vi "Connect source-meter(SubIV).vi"(8 "Error In":errorcluster, 11 "Loop data In":T2={"Persistent"={"Last file"=path "", "Last user"="", "Users"=[]}, "Temp handle"={"Connected"=FALSE, "Temp ctrl"={"Gain (P)"=0.0, "Reset (I)"=0.0, "Rate (D)"=0.0, "Stabilization rate"=0.0, "Stabilization delta"=0.0, "Type"=enum."Lake Shore 325", "Custom temp ctrl"={"VISA resource name"=""}, "Lakeshore 325"={"VISA name"="", "Loop"=0, "Heater Range"=1, "Heater Resistance"=0, "Sample sensor"=0, "Fast sensor"=0, "Slow sensor"=0}, "Lakeshore 331"={"VISA name"="", "Loop"=1, "Heater Range"=0, "Sample sensor"=0, "Fast sensor"=0, "Slow sensor"=0}, "Lakeshore 332"={"VISA name"="", "Loop"=1, "Heater Range"=0, "Sample sensor"=0, "Fast sensor"=0, "Slow sensor"=0}, "Lakeshore 335"={"VISA name"="", "Loop"=1, "Sample sensor"=0, "Fast sensor"=0, "Slow sensor"=0, "Heater Range"=0, "Output mode"=enum."Off"}, "Lakeshore 336"={"VISA name"="", "Loop"=1, "Output mode"=enum."Off", "Max current"=1.0, "Heater resistance"=1, "Sample sensor"=1, "Slow sensor"=1, "Fast sensor"=1}}}, "Paths"={"Manual"=path "", "Settings"=path "", "Persistent"=path "", "Work dir."=path ""}, "Settings"={"MFIA"={"Address"="", "Use compensation"=TRUE, "Shut down gracefully"=FALSE}, "Temp ctrl"={"Gain (P)"=0.0, "Reset (I)"=0.0, "Rate (D)"=0.0, "Stabilization rate"=0.0, "Stabilization delta"=0.0, "Type"=enum."Lake Shore 325", "Custom temp ctrl"={"VISA resource name"=""}, "Lakeshore 325"={"VISA name"="", "Loop"=0, "Heater Range"=1, "Heater Resistance"=0, "Sample sensor"=0, "Fast sensor"=0, "Slow sensor"=0}, "Lakeshore 331"={"VISA name"="", "Loop"=1, "Heater Range"=0, "Sample sensor"=0, "Fast sensor"=0, "Slow sensor"=0}, "Lakeshore 332"={"VISA name"="", "Loop"=1, "Heater Range"=0, "Sample sensor"=0, "Fast sensor"=0, "Slow sensor"=0}, "Lakeshore 335"={"VISA name"="", "Loop"=1, "Sample sensor"=0, "Fast sensor"=0, "Slow sensor"=0, "Heater Range"=0, "Output mode"=enum."Off"}, "Lakeshore 336"={"VISA name"="", "Loop"=1, "Output mode"=enum."Off", "Max current"=1.0, "Heater resistance"=1, "Sample sensor"=1, "Slow sensor"=1, "Fast sensor"=1}}, "Source-meter"={"Type"=enum."Custom", "Custom source-meter"={"VISA resource name"=""}, "Keithley 2600"={"VISA name"="", "Ignore ID Query"=FALSE, "SMU"=enum."Channel A"}, "Keithley 2400 Series"={"VISA name"="", "Ignore ID Query"=FALSE}}, "Other"={"Enable OriginLab"=FALSE, "Reader mode"=FALSE, "Auto-save"=FALSE}, "Defaults"={"IV properties"={"T"=0.0, "Vstart"=-0.5, "Vstop"=0.5, "Vpoints"=10.0, "Settling"=0.01, "I limit"=0.1, "Log mapping"=FALSE, "Averaging"=0.0}, "CV properties"={"T"=0.0, "Vstart"=-0.5, "Vstop"=0.5, "Vpoints"=10.0, "Precision"=enum."Normal", "Test signal"=0.01, "Auto I range"=FALSE, "Test frequency"=100000.0, "I range"=-2.0, "V range"=10.0, "Log mapping"=FALSE, "Rel perm"=0.0, "Area"=0.0, "Equivalent circuit model"=0}, "DLTS properties"={"Tstart"=0.0, "Instant start"=FALSE, "Tstop"=0.0, "T rate"=0.0, "Test signal"=0.0, "Test frequency"=0.0, "Bandwidth"=0.0, "Averaging"=0.0, "Vbias"=0.0, "Vpulse"=0.0, "pulse length"=0.0, "Pulse 2"=FALSE, "Vpulse 2"=0.0, "pulse length 2"=0.0, "I range"=-2.0, "V range"=10.0, "Emission rate"=[], "Sampling rate"=0.0, "Acq. delay"=0.0, "Filter order"=0, "Equivalent circuit model"=0}, "LDLTS properties"={"T"=0.0, "Test signal"=0.0, "Test frequency"=0.0, "Bandwidth"=0.0, "Averaging"=0.0, "Vbias"=0.0, "Vpulse"=0.0, "pulse length"=0.0, "Pulse 2"=FALSE, "Vpulse 2"=0.0, "pulse length 2"=0.0, "I range"=-2.0, "V range"=10.0, "Sampling rate"=0.0, "Acq. delay"=0.0, "Sampling time"=0.0, "Filter order"=0, "Equivalent circuit model"=0}}}, "Software version"=0.0, "MFIA handle"={"ziHandle"={"handleValid"=FALSE, "Conn"=0, "Path Prefix"="", "Handle"=0, "Connected"=FALSE, "Clockbase(s)"=0.0}, "Selected device"="", "ziModHandle"={"handleValid"=FALSE, "Conn"=0, "ModHandle"=0, "moduleID"="", "Path Prefix"=""}}, "Source-meter handle"={"Connected"=FALSE, "Source-meter"={"Type"=enum."Keithley 2600", "Custom source-meter"={"VISA resource name"=""}, "Keithley 2600"={"VISA name"="", "Ignore ID Query"=FALSE, "SMU"=enum."Channel A"}, "Keithley 2400 Series"={"VISA name"="", "Ignore ID Query"=FALSE}}}} {"MFIA handle"."ziModHandle"."ModHandle" format="0x%08x"; "MFIA handle"."ziModHandle"."Conn" format="0x%08x"; "MFIA handle"."ziHandle"."Handle" format="0x%08x"; "MFIA handle"."ziHandle"."Conn" format="0x%08x"; "Settings"."Defaults"."LDLTS properties"."Equivalent circuit model" items=["Rp || Cp", "Rs + Cs", "Rs + Ls", "G B", "D Cs", "Q Cs", "D Ls", "Q Ls", "Rp || Lp", "D Cp"]; "Settings"."Defaults"."LDLTS properties"."Filter order" min=0 max=8 step=1; "Settings"."Defaults"."LDLTS properties"."Sampling rate" items=["13k"=13392.857422, "27k"=26785.714844, "54k"=53571.429687, "107k"=107142.859375]; "Settings"."Defaults"."LDLTS properties"."V range" items=["10mV"=0.01, "100mV"=0.1, "1V"=1.0, "10V"=10.0]; "Settings"."Defaults"."LDLTS properties"."I range" items=["100nA"=-7.0, "1µA"=-6.0, "10µA"=-5.0, "100µA"=-4.0, "1mA"=-3.0, "10mA"=-2.0]; "Settings"."Defaults"."DLTS properties"."Equivalent circuit model" items=["Rp || Cp", "Rs + Cs", "Rs + Ls", "G B", "D Cs", "Q Cs", "D Ls", "Q Ls", "Rp || Lp", "D Cp"]; "Settings"."Defaults"."DLTS properties"."Filter order" min=0 max=8 step=1; "Settings"."Defaults"."DLTS properties"."Sampling rate" items=["13k"=13392.857422, "27k"=26785.714844, "54k"=53571.429687, "107k"=107142.859375]; "Settings"."Defaults"."DLTS properties"."V range" items=["10mV"=0.01, "100mV"=0.1, "1V"=1.0, "10V"=10.0]; "Settings"."Defaults"."DLTS properties"."I range" items=["10mV"=0.01, "100mV"=0.1, "1V"=1.0, "10V"=10.0]; "Settings"."Defaults"."CV properties"."Equivalent circuit model" items=["Rp || Cp", "Rs + Cs", "Rs + Ls", "G B", "D Cs", "Q Cs", "D Ls", "Q Ls", "Rp || Lp", "D Cp"]; "Settings"."Defaults"."CV properties"."V range" items=["10mV"=0.01, "100mV"=0.1, "1V"=1.0, "10V"=10.0]; "Settings"."Defaults"."CV properties"."I range" items=["100nA"=-7.0, "1µA"=-6.0, "10µA"=-5.0, "100µA"=-4.0, "1mA"=-3.0, "10mA"=-2.0]; "Settings"."Defaults"."IV properties"."Settling" min=0.0 max=65535.0; "Settings"."Temp ctrl"."Lakeshore 336"."Fast sensor" items=["Sensor A", "Sensor B", "Sensor C", "Sensor D"]; "Settings"."Temp ctrl"."Lakeshore 336"."Slow sensor" items=["Sensor A", "Sensor B", "Sensor C", "Sensor D"]; "Settings"."Temp ctrl"."Lakeshore 336"."Sample sensor" items=["Sensor A", "Sensor B", "Sensor C", "Sensor D"]; "Settings"."Temp ctrl"."Lakeshore 336"."Heater resistance" items=["25 Ohm"=1, "50 Ohm"=2]; "Settings"."Temp ctrl"."Lakeshore 336"."Max current" items=["0.707 A"=0.0, "1 A"=1.0, "1.414 A"=1.414, "2 A"=2.0]; "Settings"."Temp ctrl"."Lakeshore 336"."Loop" items=["Output 1"=1, "Output 2"=2, "Output 3"=3, "Output 4"=4]; "Settings"."Temp ctrl"."Lakeshore 335"."Heater Range" items=["Off", "Low (On)", "Medium", "High"]; "Settings"."Temp ctrl"."Lakeshore 335"."Slow sensor" items=["A", "B"]; "Settings"."Temp ctrl"."Lakeshore 335"."Fast sensor" items=["A", "B"]; "Settings"."Temp ctrl"."Lakeshore 335"."Sample sensor" items=["A", "B"]; "Settings"."Temp ctrl"."Lakeshore 335"."Loop" items=["Loop 1"=1, "Loop 2"=2]; "Settings"."Temp ctrl"."Lakeshore 332"."Slow sensor" items=["A", "B"]; "Settings"."Temp ctrl"."Lakeshore 332"."Fast sensor" items=["A", "B"]; "Settings"."Temp ctrl"."Lakeshore 332"."Sample sensor" items=["A", "B"]; "Settings"."Temp ctrl"."Lakeshore 332"."Heater Range" items=["Off", "Low (0.5W)", "Med (5W)", "High (50W)"]; "Settings"."Temp ctrl"."Lakeshore 332"."Loop" items=["Loop 1", "Loop 2"]; "Settings"."Temp ctrl"."Lakeshore 331"."Slow sensor" items=["A", "B"]; "Settings"."Temp ctrl"."Lakeshore 331"."Fast sensor" items=["A", "B"]; "Settings"."Temp ctrl"."Lakeshore 331"."Sample sensor" items=["A", "B"]; "Settings"."Temp ctrl"."Lakeshore 331"."Heater Range" items=["Off", "Low (0.5W)", "Med (5W)", "High (50W)"]; "Settings"."Temp ctrl"."Lakeshore 331"."Loop" items=["Loop 1", "Loop 2"]; "Settings"."Temp ctrl"."Lakeshore 325"."Slow sensor" items=["A", "B"]; "Settings"."Temp ctrl"."Lakeshore 325"."Fast sensor" items=["A", "B"]; "Settings"."Temp ctrl"."Lakeshore 325"."Sample sensor" items=["A", "B"]; "Settings"."Temp ctrl"."Lakeshore 325"."Heater Resistance" items=["25 Ohm"=1, "50 Ohm"=2]; "Settings"."Temp ctrl"."Lakeshore 325"."Heater Range" items=["Off", "Low (loop 1) or On (loop 2)", "High (loop 1)"]; "Settings"."Temp ctrl"."Lakeshore 325"."Loop" items=["Loop 1"=1, "Loop 2"=2]; "Temp handle"."Temp ctrl"."Lakeshore 336"."Fast sensor" items=["Sensor A", "Sensor B", "Sensor C", "Sensor D"]; "Temp handle"."Temp ctrl"."Lakeshore 336"."Slow sensor" items=["Sensor A", "Sensor B", "Sensor C", "Sensor D"]; "Temp handle"."Temp ctrl"."Lakeshore 336"."Sample sensor" items=["Sensor A", "Sensor B", "Sensor C", "Sensor D"]; "Temp handle"."Temp ctrl"."Lakeshore 336"."Heater resistance" items=["25 Ohm"=1, "50 Ohm"=2]; "Temp handle"."Temp ctrl"."Lakeshore 336"."Max current" items=["0.707 A"=0.0, "1 A"=1.0, "1.414 A"=1.414, "2 A"=2.0]; "Temp handle"."Temp ctrl"."Lakeshore 336"."Loop" items=["Output 1"=1, "Output 2"=2, "Output 3"=3, "Output 4"=4]; "Temp handle"."Temp ctrl"."Lakeshore 335"."Heater Range" items=["Off", "Low (On)", "Medium", "High"]; "Temp handle"."Temp ctrl"."Lakeshore 335"."Slow sensor" items=["A", "B"]; "Temp handle"."Temp ctrl"."Lakeshore 335"."Fast sensor" items=["A", "B"]; "Temp handle"."Temp ctrl"."Lakeshore 335"."Sample sensor" items=["A", "B"]; "Temp handle"."Temp ctrl"."Lakeshore 335"."Loop" items=["Loop 1"=1, "Loop 2"=2]; "Temp handle"."Temp ctrl"."Lakeshore 332"."Slow sensor" items=["A", "B"]; "Temp handle"."Temp ctrl"."Lakeshore 332"."Fast sensor" items=["A", "B"]; "Temp handle"."Temp ctrl"."Lakeshore 332"."Sample sensor" items=["A", "B"]; "Temp handle"."Temp ctrl"."Lakeshore 332"."Heater Range" items=["Off", "Low (0.5W)", "Med (5W)", "High (50W)"]; "Temp handle"."Temp ctrl"."Lakeshore 332"."Loop" items=["Loop 1", "Loop 2"]; "Temp handle"."Temp ctrl"."Lakeshore 331"."Slow sensor" items=["A", "B"]; "Temp handle"."Temp ctrl"."Lakeshore 331"."Fast sensor" items=["A", "B"]; "Temp handle"."Temp ctrl"."Lakeshore 331"."Sample sensor" items=["A", "B"]; "Temp handle"."Temp ctrl"."Lakeshore 331"."Heater Range" items=["Off", "Low (0.5W)", "Med (5W)", "High (50W)"]; "Temp handle"."Temp ctrl"."Lakeshore 331"."Loop" items=["Loop 1", "Loop 2"]; "Temp handle"."Temp ctrl"."Lakeshore 325"."Slow sensor" items=["A", "B"]; "Temp handle"."Temp ctrl"."Lakeshore 325"."Fast sensor" items=["A", "B"]; "Temp handle"."Temp ctrl"."Lakeshore 325"."Sample sensor" items=["A", "B"]; "Temp handle"."Temp ctrl"."Lakeshore 325"."Heater Resistance" items=["25 Ohm"=1, "50 Ohm"=2]; "Temp handle"."Temp ctrl"."Lakeshore 325"."Heater Range" items=["Off", "Low (loop 1) or On (loop 2)", "High (loop 1)"]; "Temp handle"."Temp ctrl"."Lakeshore 325"."Loop" items=["Loop 1"=1, "Loop 2"=2]}) -> (0 "Error Out":errorcluster, 2 "Result":T1(ring), 3 "Loop data Out":T2={"Persistent"={"Last file"=path "", "Last user"="", "Users"=[]}, "Temp handle"={"Connected"=FALSE, "Temp ctrl"={"Gain (P)"=0.0, "Reset (I)"=0.0, "Rate (D)"=0.0, "Stabilization rate"=0.0, "Stabilization delta"=0.0, "Type"=enum."Lake Shore 325", "Custom temp ctrl"={"VISA resource name"=""}, "Lakeshore 325"={"VISA name"="", "Loop"=0, "Heater Range"=1, "Heater Resistance"=0, "Sample sensor"=0, "Fast sensor"=0, "Slow sensor"=0}, "Lakeshore 331"={"VISA name"="", "Loop"=1, "Heater Range"=0, "Sample sensor"=0, "Fast sensor"=0, "Slow sensor"=0}, "Lakeshore 332"={"VISA name"="", "Loop"=1, "Heater Range"=0, "Sample sensor"=0, "Fast sensor"=0, "Slow sensor"=0}, "Lakeshore 335"={"VISA name"="", "Loop"=1, "Sample sensor"=0, "Fast sensor"=0, "Slow sensor"=0, "Heater Range"=0, "Output mode"=enum."Off"}, "Lakeshore 336"={"VISA name"="", "Loop"=1, "Output mode"=enum."Off", "Max current"=1.0, "Heater resistance"=1, "Sample sensor"=1, "Slow sensor"=1, "Fast sensor"=1}}}, "Paths"={"Manual"=path "", "Settings"=path "", "Persistent"=path "", "Work dir."=path ""}, "Settings"={"MFIA"={"Address"="", "Use compensation"=TRUE, "Shut down gracefully"=FALSE}, "Temp ctrl"={"Gain (P)"=0.0, "Reset (I)"=0.0, "Rate (D)"=0.0, "Stabilization rate"=0.0, "Stabilization delta"=0.0, "Type"=enum."Lake Shore 325", "Custom temp ctrl"={"VISA resource name"=""}, "Lakeshore 325"={"VISA name"="", "Loop"=0, "Heater Range"=1, "Heater Resistance"=0, "Sample sensor"=0, "Fast sensor"=0, "Slow sensor"=0}, "Lakeshore 331"={"VISA name"="", "Loop"=1, "Heater Range"=0, "Sample sensor"=0, "Fast sensor"=0, "Slow sensor"=0}, "Lakeshore 332"={"VISA name"="", "Loop"=1, "Heater Range"=0, "Sample sensor"=0, "Fast sensor"=0, "Slow sensor"=0}, "Lakeshore 335"={"VISA name"="", "Loop"=1, "Sample sensor"=0, "Fast sensor"=0, "Slow sensor"=0, "Heater Range"=0, "Output mode"=enum."Off"}, "Lakeshore 336"={"VISA name"="", "Loop"=1, "Output mode"=enum."Off", "Max current"=1.0, "Heater resistance"=1, "Sample sensor"=1, "Slow sensor"=1, "Fast sensor"=1}}, "Source-meter"={"Type"=enum."Custom", "Custom source-meter"={"VISA resource name"=""}, "Keithley 2600"={"VISA name"="", "Ignore ID Query"=FALSE, "SMU"=enum."Channel A"}, "Keithley 2400 Series"={"VISA name"="", "Ignore ID Query"=FALSE}}, "Other"={"Enable OriginLab"=FALSE, "Reader mode"=FALSE, "Auto-save"=FALSE}, "Defaults"={"IV properties"={"T"=0.0, "Vstart"=-0.5, "Vstop"=0.5, "Vpoints"=10.0, "Settling"=0.01, "I limit"=0.1, "Log mapping"=FALSE, "Averaging"=0.0}, "CV properties"={"T"=0.0, "Vstart"=-0.5, "Vstop"=0.5, "Vpoints"=10.0, "Precision"=enum."Normal", "Test signal"=0.01, "Auto I range"=FALSE, "Test frequency"=100000.0, "I range"=-2.0, "V range"=10.0, "Log mapping"=FALSE, "Rel perm"=0.0, "Area"=0.0, "Equivalent circuit model"=0}, "DLTS properties"={"Tstart"=0.0, "Instant start"=FALSE, "Tstop"=0.0, "T rate"=0.0, "Test signal"=0.0, "Test frequency"=0.0, "Bandwidth"=0.0, "Averaging"=0.0, "Vbias"=0.0, "Vpulse"=0.0, "pulse length"=0.0, "Pulse 2"=FALSE, "Vpulse 2"=0.0, "pulse length 2"=0.0, "I range"=-2.0, "V range"=10.0, "Emission rate"=[], "Sampling rate"=0.0, "Acq. delay"=0.0, "Filter order"=0, "Equivalent circuit model"=0}, "LDLTS properties"={"T"=0.0, "Test signal"=0.0, "Test frequency"=0.0, "Bandwidth"=0.0, "Averaging"=0.0, "Vbias"=0.0, "Vpulse"=0.0, "pulse length"=0.0, "Pulse 2"=FALSE, "Vpulse 2"=0.0, "pulse length 2"=0.0, "I range"=-2.0, "V range"=10.0, "Sampling rate"=0.0, "Acq. delay"=0.0, "Sampling time"=0.0, "Filter order"=0, "Equivalent circuit model"=0}}}, "Software version"=0.0, "MFIA handle"={"ziHandle"={"handleValid"=FALSE, "Conn"=0, "Path Prefix"="", "Handle"=0, "Connected"=FALSE, "Clockbase(s)"=0.0}, "Selected device"="", "ziModHandle"={"handleValid"=FALSE, "Conn"=0, "ModHandle"=0, "moduleID"="", "Path Prefix"=""}}, "Source-meter handle"={"Connected"=FALSE, "Source-meter"={"Type"=enum."Keithley 2600", "Custom source-meter"={"VISA resource name"=""}, "Keithley 2600"={"VISA name"="", "Ignore ID Query"=FALSE, "SMU"=enum."Channel A"}, "Keithley 2400 Series"={"VISA name"="", "Ignore ID Query"=FALSE}}}} {"MFIA handle"."ziModHandle"."ModHandle" format="0x%08x"; "MFIA handle"."ziModHandle"."Conn" format="0x%08x"; "MFIA handle"."ziHandle"."Handle" format="0x%08x"; "MFIA handle"."ziHandle"."Conn" format="0x%08x"; "Settings"."Defaults"."LDLTS properties"."Equivalent circuit model" items=["Rp || Cp", "Rs + Cs", "Rs + Ls", "G B", "D Cs", "Q Cs", "D Ls", "Q Ls", "Rp || Lp", "D Cp"]; "Settings"."Defaults"."LDLTS properties"."Filter order" min=0 max=8 step=1; "Settings"."Defaults"."LDLTS properties"."Sampling rate" items=["13k"=13392.857422, "27k"=26785.714844, "54k"=53571.429687, "107k"=107142.859375]; "Settings"."Defaults"."LDLTS properties"."V range" items=["10mV"=0.01, "100mV"=0.1, "1V"=1.0, "10V"=10.0]; "Settings"."Defaults"."LDLTS properties"."I range" items=["100nA"=-7.0, "1µA"=-6.0, "10µA"=-5.0, "100µA"=-4.0, "1mA"=-3.0, "10mA"=-2.0]; "Settings"."Defaults"."DLTS properties"."Equivalent circuit model" items=["Rp || Cp", "Rs + Cs", "Rs + Ls", "G B", "D Cs", "Q Cs", "D Ls", "Q Ls", "Rp || Lp", "D Cp"]; "Settings"."Defaults"."DLTS properties"."Filter order" min=0 max=8 step=1; "Settings"."Defaults"."DLTS properties"."Sampling rate" items=["13k"=13392.857422, "27k"=26785.714844, "54k"=53571.429687, "107k"=107142.859375]; "Settings"."Defaults"."DLTS properties"."V range" items=["10mV"=0.01, "100mV"=0.1, "1V"=1.0, "10V"=10.0]; "Settings"."Defaults"."DLTS properties"."I range" items=["10mV"=0.01, "100mV"=0.1, "1V"=1.0, "10V"=10.0]; "Settings"."Defaults"."CV properties"."Equivalent circuit model" items=["Rp || Cp", "Rs + Cs", "Rs + Ls", "G B", "D Cs", "Q Cs", "D Ls", "Q Ls", "Rp || Lp", "D Cp"]; "Settings"."Defaults"."CV properties"."V range" items=["10mV"=0.01, "100mV"=0.1, "1V"=1.0, "10V"=10.0]; "Settings"."Defaults"."CV properties"."I range" items=["100nA"=-7.0, "1µA"=-6.0, "10µA"=-5.0, "100µA"=-4.0, "1mA"=-3.0, "10mA"=-2.0]; "Settings"."Defaults"."IV properties"."Settling" min=0.0 max=65535.0; "Settings"."Temp ctrl"."Lakeshore 336"."Fast sensor" items=["Sensor A", "Sensor B", "Sensor C", "Sensor D"]; "Settings"."Temp ctrl"."Lakeshore 336"."Slow sensor" items=["Sensor A", "Sensor B", "Sensor C", "Sensor D"]; "Settings"."Temp ctrl"."Lakeshore 336"."Sample sensor" items=["Sensor A", "Sensor B", "Sensor C", "Sensor D"]; "Settings"."Temp ctrl"."Lakeshore 336"."Heater resistance" items=["25 Ohm"=1, "50 Ohm"=2]; "Settings"."Temp ctrl"."Lakeshore 336"."Max current" items=["0.707 A"=0.0, "1 A"=1.0, "1.414 A"=1.414, "2 A"=2.0]; "Settings"."Temp ctrl"."Lakeshore 336"."Loop" items=["Output 1"=1, "Output 2"=2, "Output 3"=3, "Output 4"=4]; "Settings"."Temp ctrl"."Lakeshore 335"."Heater Range" items=["Off", "Low (On)", "Medium", "High"]; "Settings"."Temp ctrl"."Lakeshore 335"."Slow sensor" items=["A", "B"]; "Settings"."Temp ctrl"."Lakeshore 335"."Fast sensor" items=["A", "B"]; "Settings"."Temp ctrl"."Lakeshore 335"."Sample sensor" items=["A", "B"]; "Settings"."Temp ctrl"."Lakeshore 335"."Loop" items=["Loop 1"=1, "Loop 2"=2]; "Settings"."Temp ctrl"."Lakeshore 332"."Slow sensor" items=["A", "B"]; "Settings"."Temp ctrl"."Lakeshore 332"."Fast sensor" items=["A", "B"]; "Settings"."Temp ctrl"."Lakeshore 332"."Sample sensor" items=["A", "B"]; "Settings"."Temp ctrl"."Lakeshore 332"."Heater Range" items=["Off", "Low (0.5W)", "Med (5W)", "High (50W)"]; "Settings"."Temp ctrl"."Lakeshore 332"."Loop" items=["Loop 1", "Loop 2"]; "Settings"."Temp ctrl"."Lakeshore 331"."Slow sensor" items=["A", "B"]; "Settings"."Temp ctrl"."Lakeshore 331"."Fast sensor" items=["A", "B"]; "Settings"."Temp ctrl"."Lakeshore 331"."Sample sensor" items=["A", "B"]; "Settings"."Temp ctrl"."Lakeshore 331"."Heater Range" items=["Off", "Low (0.5W)", "Med (5W)", "High (50W)"]; "Settings"."Temp ctrl"."Lakeshore 331"."Loop" items=["Loop 1", "Loop 2"]; "Settings"."Temp ctrl"."Lakeshore 325"."Slow sensor" items=["A", "B"]; "Settings"."Temp ctrl"."Lakeshore 325"."Fast sensor" items=["A", "B"]; "Settings"."Temp ctrl"."Lakeshore 325"."Sample sensor" items=["A", "B"]; "Settings"."Temp ctrl"."Lakeshore 325"."Heater Resistance" items=["25 Ohm"=1, "50 Ohm"=2]; "Settings"."Temp ctrl"."Lakeshore 325"."Heater Range" items=["Off", "Low (loop 1) or On (loop 2)", "High (loop 1)"]; "Settings"."Temp ctrl"."Lakeshore 325"."Loop" items=["Loop 1"=1, "Loop 2"=2]; "Temp handle"."Temp ctrl"."Lakeshore 336"."Fast sensor" items=["Sensor A", "Sensor B", "Sensor C", "Sensor D"]; "Temp handle"."Temp ctrl"."Lakeshore 336"."Slow sensor" items=["Sensor A", "Sensor B", "Sensor C", "Sensor D"]; "Temp handle"."Temp ctrl"."Lakeshore 336"."Sample sensor" items=["Sensor A", "Sensor B", "Sensor C", "Sensor D"]; "Temp handle"."Temp ctrl"."Lakeshore 336"."Heater resistance" items=["25 Ohm"=1, "50 Ohm"=2]; "Temp handle"."Temp ctrl"."Lakeshore 336"."Max current" items=["0.707 A"=0.0, "1 A"=1.0, "1.414 A"=1.414, "2 A"=2.0]; "Temp handle"."Temp ctrl"."Lakeshore 336"."Loop" items=["Output 1"=1, "Output 2"=2, "Output 3"=3, "Output 4"=4]; "Temp handle"."Temp ctrl"."Lakeshore 335"."Heater Range" items=["Off", "Low (On)", "Medium", "High"]; "Temp handle"."Temp ctrl"."Lakeshore 335"."Slow sensor" items=["A", "B"]; "Temp handle"."Temp ctrl"."Lakeshore 335"."Fast sensor" items=["A", "B"]; "Temp handle"."Temp ctrl"."Lakeshore 335"."Sample sensor" items=["A", "B"]; "Temp handle"."Temp ctrl"."Lakeshore 335"."Loop" items=["Loop 1"=1, "Loop 2"=2]; "Temp handle"."Temp ctrl"."Lakeshore 332"."Slow sensor" items=["A", "B"]; "Temp handle"."Temp ctrl"."Lakeshore 332"."Fast sensor" items=["A", "B"]; "Temp handle"."Temp ctrl"."Lakeshore 332"."Sample sensor" items=["A", "B"]; "Temp handle"."Temp ctrl"."Lakeshore 332"."Heater Range" items=["Off", "Low (0.5W)", "Med (5W)", "High (50W)"]; "Temp handle"."Temp ctrl"."Lakeshore 332"."Loop" items=["Loop 1", "Loop 2"]; "Temp handle"."Temp ctrl"."Lakeshore 331"."Slow sensor" items=["A", "B"]; "Temp handle"."Temp ctrl"."Lakeshore 331"."Fast sensor" items=["A", "B"]; "Temp handle"."Temp ctrl"."Lakeshore 331"."Sample sensor" items=["A", "B"]; "Temp handle"."Temp ctrl"."Lakeshore 331"."Heater Range" items=["Off", "Low (0.5W)", "Med (5W)", "High (50W)"]; "Temp handle"."Temp ctrl"."Lakeshore 331"."Loop" items=["Loop 1", "Loop 2"]; "Temp handle"."Temp ctrl"."Lakeshore 325"."Slow sensor" items=["A", "B"]; "Temp handle"."Temp ctrl"."Lakeshore 325"."Fast sensor" items=["A", "B"]; "Temp handle"."Temp ctrl"."Lakeshore 325"."Sample sensor" items=["A", "B"]; "Temp handle"."Temp ctrl"."Lakeshore 325"."Heater Resistance" items=["25 Ohm"=1, "50 Ohm"=2]; "Temp handle"."Temp ctrl"."Lakeshore 325"."Heater Range" items=["Off", "Low (loop 1) or On (loop 2)", "High (loop 1)"]; "Temp handle"."Temp ctrl"."Lakeshore 325"."Loop" items=["Loop 1"=1, "Loop 2"=2]})   [LabVIEW 2019]
doc: "Handles connection to a source-meter"
uses:
  Type defs/Loop data Type Def.ctl
  Type defs/Persistent Type Def.ctl
  Type defs/Temp handle Type Def.ctl
  Type defs/Temp ctrl Type Def.ctl
  Custom devices/Custom temp ctrl settings.ctl
  Type defs/Paths Type Def.ctl
  Type defs/Settings Type Def.ctl
  Type defs/Imps Type Def.ctl
  Type defs/Source-meter Type Def.ctl
  Custom devices/Custom source-meter settings.ctl
  Type defs/Other settings Type Def.ctl
  Type defs/IV properties Type Def.ctl
  Type defs/CV properties Type Def.ctl
  Type defs/DLTS properties Type Def.ctl
  Type defs/LDLTS properties Type Def.ctl
  Type defs/MFIA handle Type Def.ctl
  <instrlib>/Zurich Instruments LabOne/Public/ziTypeHandle.ctl
  <instrlib>/Zurich Instruments LabOne/Public/Modules/ziTypeModHandle.ctl
  Type defs/Source-meter handle Type Def.ctl
  <instrlib>/Keithley 2600 Series/Keithley 2600 Series.lvlib
  <instrlib>/Keithley 2450/Keithley 2450.lvlib
  <instrlib>/Zurich Instruments LabOne/Zurich Instruments LabOne.lvlib
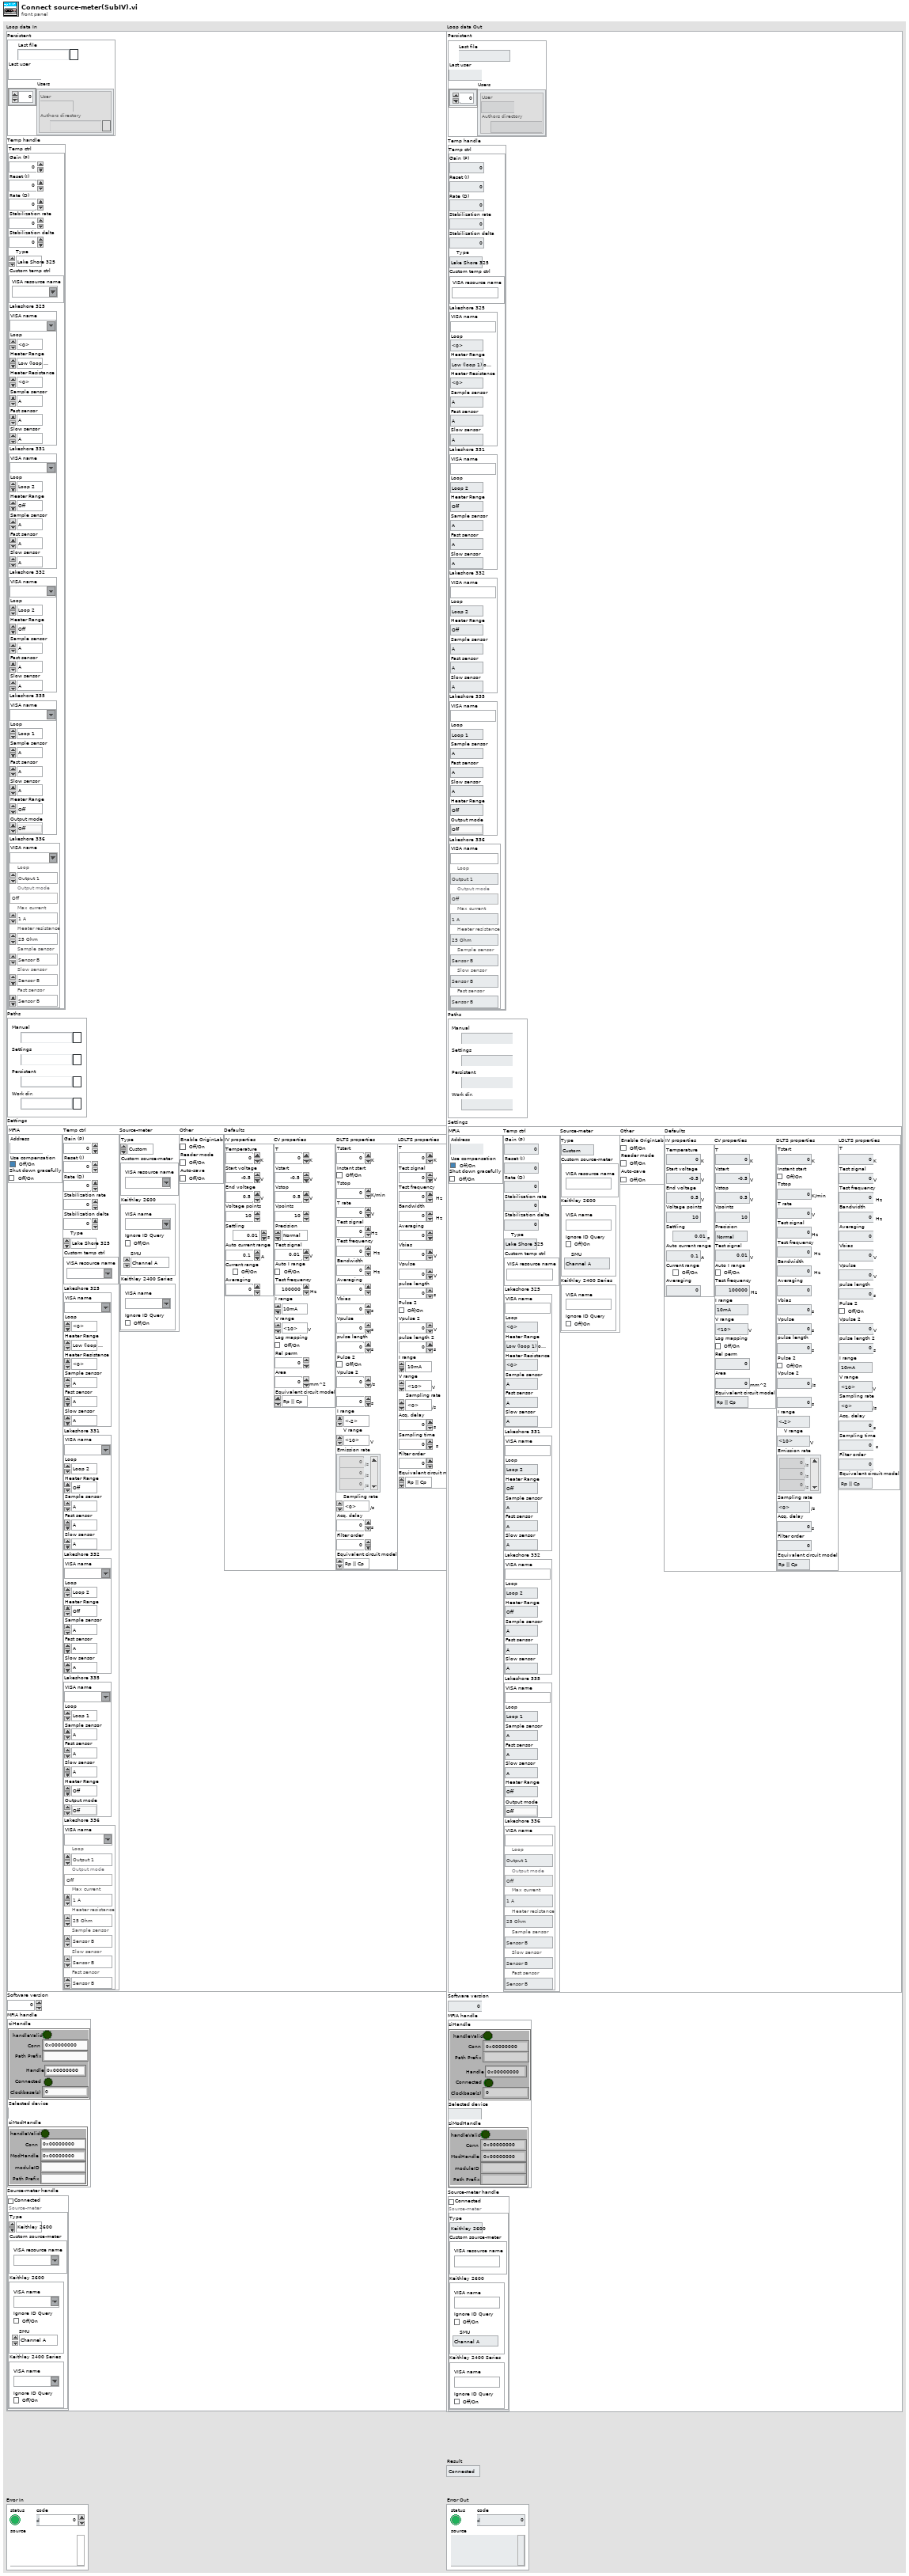
[diagram p1: front panel]
types:
  T1 = enum16{"Connected", "Not connected", "Incorrect settings"}
  T2 = typedef "Loop data Type Def.ctl" = cluster{"Persistent":T3, "Temp handle":T4, "Paths":T7, "Settings":T8, "Software version":dbl, "MFIA handle":T17, "Source-meter handle":T20}
  T3 = typedef "Persistent Type Def.ctl" = cluster{"Last file":path, "Last user":string, "Users":cluster{"User":string, "Authors directory":path}[]}
  T4 = typedef "Temp handle Type Def.ctl" = cluster{"Connected":bool, "Temp ctrl":T5}
  T5 = typedef "Temp ctrl Type Def.ctl" = cluster{"Gain (P)":dbl, "Reset (I)":dbl, "Rate (D)":dbl, "Stabilization rate":dbl, "Stabilization delta":dbl, "Type":enum16{"Custom", "Lake Shore 325", "Lake Shore 331", "Lake Shore 332", "Lake Shore 335", "Lake Shore 336"}, "Custom temp ctrl":T6, "Lakeshore 325":cluster{"VISA name":refnum<visa-resource-name>, "Loop":u16, "Heater Range":u16, "Heater Resistance":u16, "Sample sensor":u16, "Fast sensor":u16, "Slow sensor":u16}, "Lakeshore 331":cluster{"VISA name":refnum<visa-resource-name>, "Loop":u16, "Heater Range":u16, "Sample sensor":u16, "Fast sensor":u16, "Slow sensor":u16}, "Lakeshore 332":cluster{"VISA name":refnum<visa-resource-name>, "Loop":u16, "Heater Range":u16, "Sample sensor":u16, "Fast sensor":u16, "Slow sensor":u16}, "Lakeshore 335":cluster{"VISA name":refnum<visa-resource-name>, "Loop":u16, "Sample sensor":u16, "Fast sensor":u16, "Slow sensor":u16, "Heater Range":u16, "Output mode":enum16{"Off", "Closed Loop PID", "Zone", "Open Loop", "Monitor Out", "Warmup Supply"}}, "Lakeshore 336":cluster{"VISA name":refnum<visa-resource-name>, "Loop":u16, "Output mode":enum16{"Off", "Closed Loop PID", "Zone", "Open Loop"}, "Max current":dbl, "Heater resistance":u16, "Sample sensor":u16, "Slow sensor":u16, "Fast sensor":u16}}
  T6 = typedef "Custom temp ctrl settings.ctl" = cluster{"VISA resource name":refnum<visa-resource-name>}
  T7 = typedef "Paths Type Def.ctl" = cluster{"Manual":path, "Settings":path, "Persistent":path, "Work dir.":path}
  T8 = typedef "Settings Type Def.ctl" = cluster{"MFIA":T9, "Temp ctrl":T5, "Source-meter":T10, "Other":T12, "Defaults":cluster{"IV properties":T13, "CV properties":T14, "DLTS properties":T15, "LDLTS properties":T16}}
  T9 = typedef "Imps Type Def.ctl" = cluster{"Address":string, "Use compensation":bool, "Shut down gracefully":bool}
  T10 = typedef "Source-meter Type Def.ctl" = cluster{"Type":enum16{"Custom", "Keithley 2600", "Keithley 2400 Series"}, "Custom source-meter":T11, "Keithley 2600":cluster{"VISA name":refnum<visa-resource-name>, "Ignore ID Query":bool, "SMU":enum16{"Channel A", "Channel B"}}, "Keithley 2400 Series":cluster{"VISA name":refnum<visa-resource-name>, "Ignore ID Query":bool}}
  T11 = typedef "Custom source-meter settings.ctl" = cluster{"VISA resource name":refnum<visa-resource-name>}
  T12 = typedef "Other settings Type Def.ctl" = cluster{"Enable OriginLab":bool, "Reader mode":bool, "Auto-save":bool}
  T13 = typedef "IV properties Type Def.ctl" = cluster{"T":dbl[unit], "Vstart":dbl[unit], "Vstop":dbl[unit], "Vpoints":dbl, "Settling":dbl[unit], "I limit":dbl[unit], "Log mapping":bool, "Averaging":dbl}
  T14 = typedef "CV properties Type Def.ctl" = cluster{"T":dbl[unit], "Vstart":dbl[unit], "Vstop":dbl[unit], "Vpoints":dbl, "Precision":enum16{"Low (Fast)", "Normal", "High (Slow)"}, "Test signal":dbl[unit], "Auto I range":bool, "Test frequency":dbl[unit], "I range":dbl, "V range":dbl[unit], "Log mapping":bool, "Rel perm":dbl, "Area":dbl[unit], "Equivalent circuit model":u16}
  T15 = typedef "DLTS properties Type Def.ctl" = cluster{"Tstart":dbl[unit], "Instant start":bool, "Tstop":dbl[unit], "T rate":dbl[unit], "Test signal":dbl[unit], "Test frequency":dbl[unit], "Bandwidth":dbl[unit], "Averaging":dbl, "Vbias":dbl[unit], "Vpulse":dbl[unit], "pulse length":dbl[unit], "Pulse 2":bool, "Vpulse 2":dbl[unit], "pulse length 2":dbl[unit], "I range":dbl, "V range":dbl[unit], "Emission rate":dbl[unit][], "Sampling rate":dbl[unit], "Acq. delay":dbl[unit], "Filter order":i32, "Equivalent circuit model":u16}
  T16 = typedef "LDLTS properties Type Def.ctl" = cluster{"T":dbl[unit], "Test signal":dbl[unit], "Test frequency":dbl[unit], "Bandwidth":dbl[unit], "Averaging":dbl, "Vbias":dbl[unit], "Vpulse":dbl[unit], "pulse length":dbl[unit], "Pulse 2":bool, "Vpulse 2":dbl[unit], "pulse length 2":dbl[unit], "I range":dbl, "V range":dbl[unit], "Sampling rate":dbl[unit], "Acq. delay":dbl[unit], "Sampling time":dbl[unit], "Filter order":i32, "Equivalent circuit model":u16}
  T17 = typedef "MFIA handle Type Def.ctl" = cluster{"ziHandle":T18, "Selected device":string, "ziModHandle":T19}
  T18 = typedef "Zurich Instruments LabOne.lvlib/ziTypeHandle.ctl" = cluster{"handleValid":bool, "Conn":u64, "Path Prefix":string, "Handle":u64, "Connected":bool, "Clockbase(s)":dbl}
  T19 = typedef "Zurich Instruments LabOne.lvlib/ziTypeModHandle.ctl" = cluster{"handleValid":bool, "Conn":u64, "ModHandle":u64, "moduleID":string, "Path Prefix":string}
  T20 = typedef "Source-meter handle Type Def.ctl" = cluster{"Connected":bool, "Source-meter":T10}
  T21 = enum16{"Custom", "Keithley 2600", "Keithley 2400 Series"}
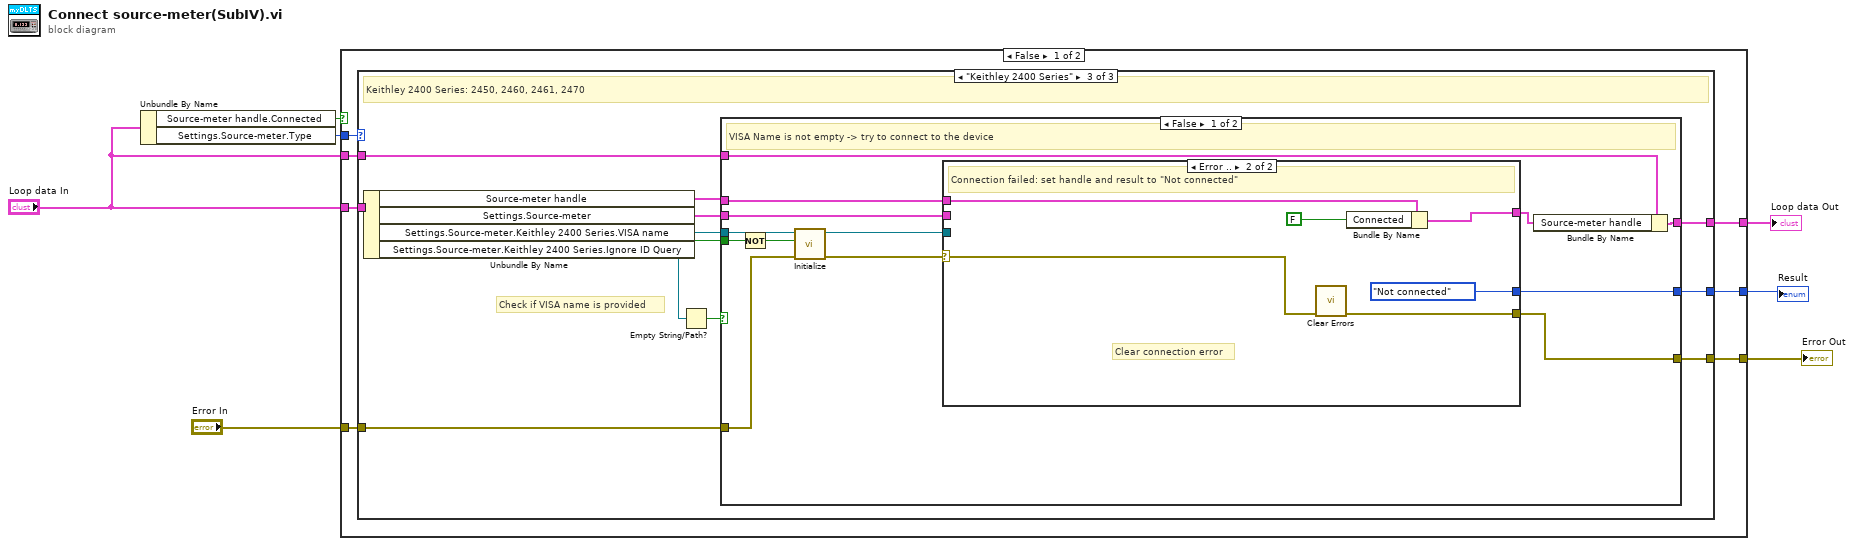
[diagram p0: block diagram]
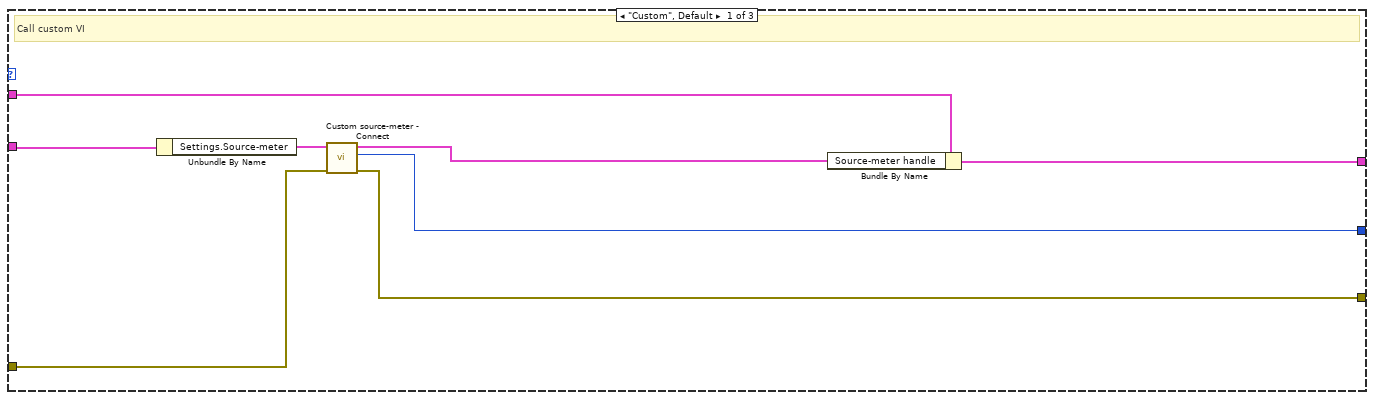
[diagram p2: hidden frame]
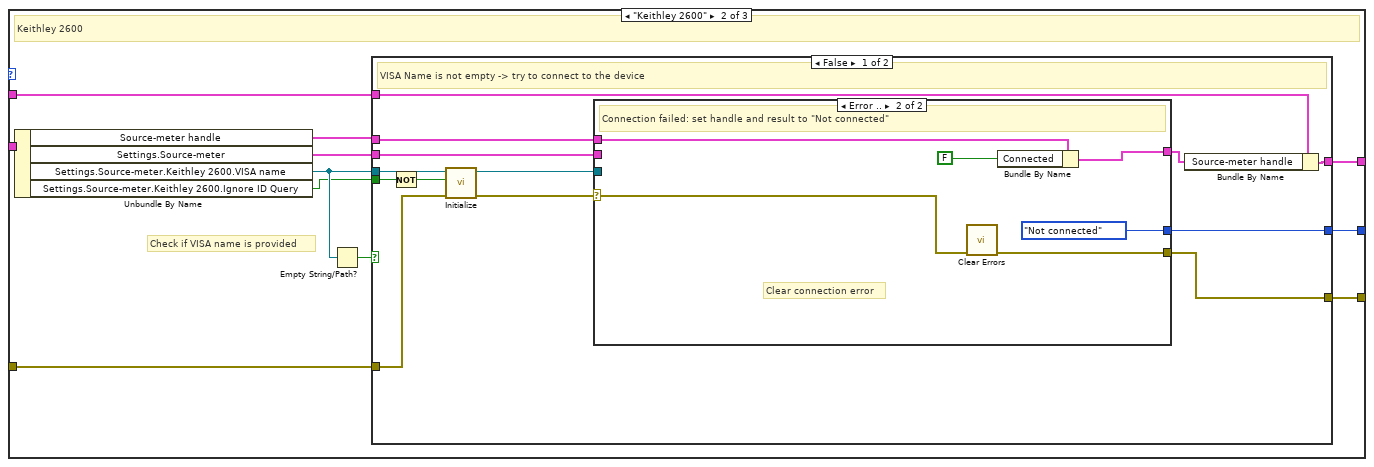
[diagram p3: hidden frame]
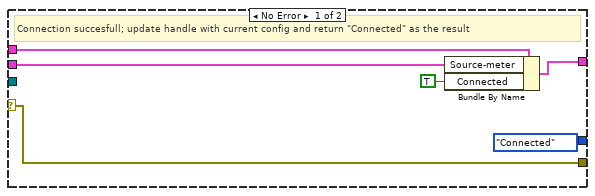
[diagram p4: hidden frame]
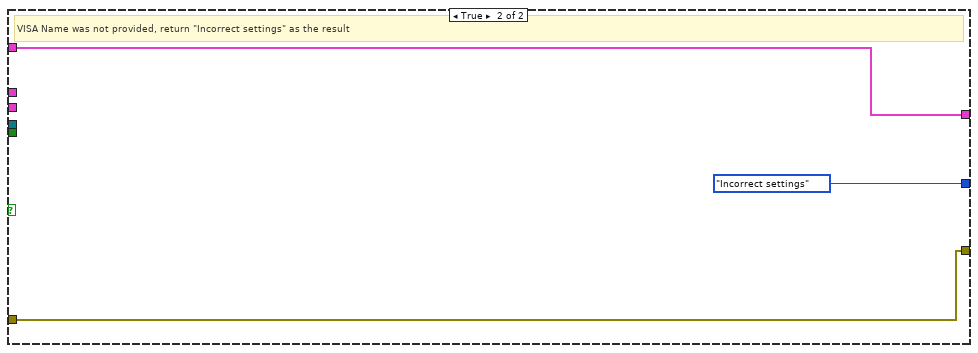
[diagram p5: hidden frame]
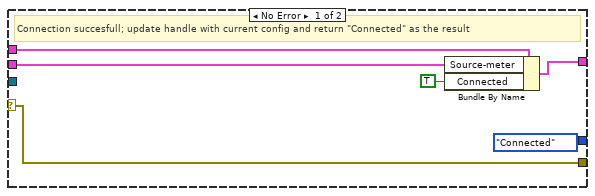
[diagram p6: hidden frame]
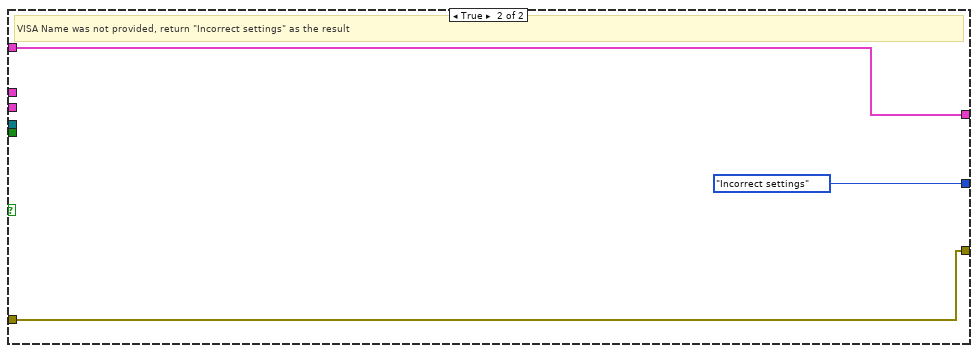
[diagram p7: hidden frame]
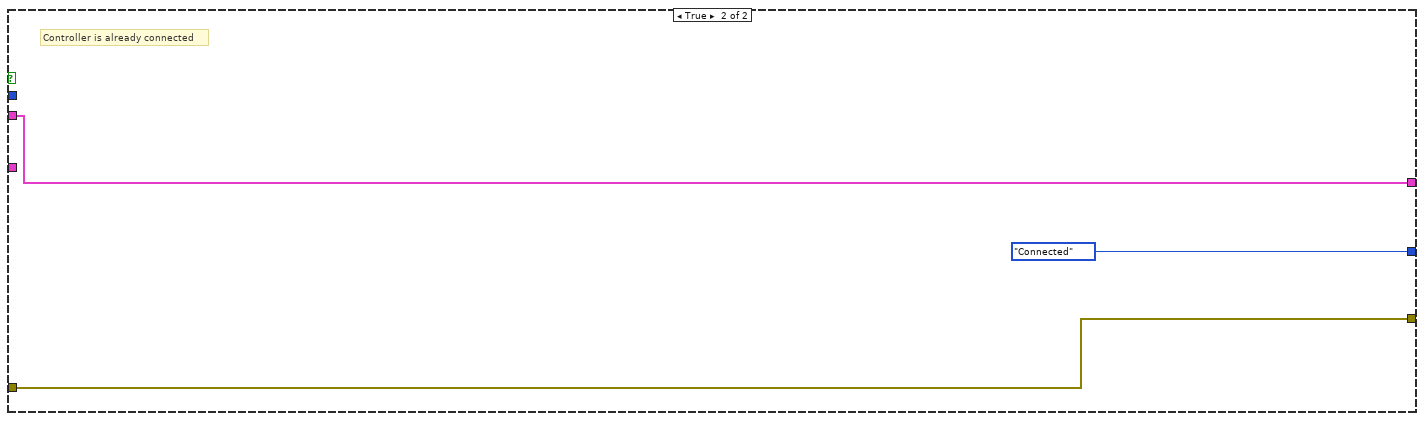
[diagram p8: hidden frame]
diagram:
  n1 = Unbundle By Name("Loop data In") -> ("Source-meter handle.Connected"=w3:bool, "Settings.Source-meter.Type"=w2:T21)
  n2 = case shown="False" w3 {
    tunnel: [w14 w102] -> w7
    tunnel: [w13 T1."Connected" ("Result")] -> w6
    tunnel: "Error In" -> [w12 w101]
    tunnel: "Loop data In" -> [w11 w102]
    tunnel: [w10 w101] -> w4
    tunnel: w2 -> [w9 _]
    tunnel: "Loop data In" -> [w8 _]
    frame False {
      n3 = case shown="\"Keithley 2400 Series\"" w9 {
        tunnel: [w20 w31 w70] -> w14
        tunnel: [w16 w33 w72] -> w13
        tunnel: w12 -> [w18 w30 w69]
        tunnel: w11 -> [w21 w29 w68]
        tunnel: [w17 w28 w67] -> w10
        tunnel: w8 -> [w22 w27 w66]
        frame "Custom", Default {
          # "Call custom VI"
          n4 = Unbundle By Name(w22) -> ("Settings.Source-meter"=w19:T10)
          n5 = call "Custom source-meter - Connect.vi"("Error In"=w18, "Source-meter"=w19) -> ("Error Out"=w17:errorcluster, "Result"=w16:T1, "Source-meter handle"=w15:T20)  [unwired: 7 in]
          n6 = Bundle By Name(cluster=w21, "Source-meter handle"=w15) -> (w20:T2)
        }
        frame "Keithley 2600" {
          # "Check if VISA name is provided"
          # "Keithley 2600"
          n7 = Unbundle By Name(w27) -> ("Source-meter handle"=w26:T20, "Settings.Source-meter"=w24:T10, "Settings.Source-meter.Keithley 2600.VISA name"=w25:refnum<visa-resource-name>, "Settings.Source-meter.Keithley 2600.Ignore ID Query"=w23:bool)
          n8 = Empty String/Path?(string/path=w25) -> (empty?=w32:bool)
          n9 = case shown="False" w32 {
            tunnel: [w45 T1."Incorrect settings" ("Result")] -> w33
            tunnel: [w42 w60] -> w31
            tunnel: w25 -> [w36 _]
            tunnel: w30 -> [w39 w59]
            tunnel: w26 -> [w46 _]
            tunnel: w29 -> [w44 w60]
            tunnel: [w41 w59] -> w28
            tunnel: w24 -> [w40 _]
            tunnel: w23 -> [w35 _]
            frame False {
              # "VISA Name is not empty -> try to connect to the device"
              n10 = Not(x=w35) -> (.not. x?=w34:bool)
              n11 = call <instrlib>:"Initialize.vi"("error in (no error)"=w39, "ID Query (True)"=w34, "VISA resource name"=w36) -> ("error out"=w38:errorcluster, "VISA resource name out"=w37:refnum<visa-resource-name>)  [unwired: 7 in]
              n12 = case shown="Error .." w38 {
                selector: w38 -> [w48 w55]
                tunnel: w37 -> [_ _]
                tunnel: [w48 w54] -> w41
                tunnel: w46 -> [w51 w57]
                tunnel: [w52 w56] -> w43
                tunnel: [T1."Connected" ("Result") T1."Not connected" ("Result")] -> w45
                tunnel: w40 -> [w47 _]
                frame No Error {
                  # "Connection succesfull; update handle with current config and return \"Connected\" as the result"
                  n13 = Bundle By Name(cluster=w51, "Source-meter"=w47, "Connected"=TRUE) -> (w52:T20)
                }
                frame Error {
                  # "Clear connection error"
                  # "Connection failed: set handle and result to \"Not connected\""
                  n14 = call <vilib>:"Clear Errors.vi"("error in (no error)"=w55) -> ("error out"=w54:errorcluster)  [unwired: 5 in, 1 out]
                  n15 = Bundle By Name(cluster=w57, "Connected"=FALSE ("Temp handle.Connected")) -> (w56:T20)
                }
              }
              n16 = Bundle By Name(cluster=w44, "Source-meter handle"=w43) -> (w42:T2)
            }
            frame True {
              # "VISA Name was not provided, return \"Incorrect settings\" as the result"
            }
          }
        }
        frame "Keithley 2400 Series" {
          # "Check if VISA name is provided"
          # "Keithley 2400 Series: 2450, 2460, 2461, 2470"
          n17 = Unbundle By Name(w66) -> ("Source-meter handle"=w65:T20, "Settings.Source-meter"=w63:T10, "Settings.Source-meter.Keithley 2400 Series.VISA name"=w64:refnum<visa-resource-name>, "Settings.Source-meter.Keithley 2400 Series.Ignore ID Query"=w62:bool)
          n18 = Empty String/Path?(string/path=w64) -> (empty?=w71:bool)
          n19 = case shown="False" w71 {
            tunnel: [w84 T1."Incorrect settings" ("Result")] -> w72
            tunnel: [w81 w99] -> w70
            tunnel: w64 -> [w75 _]
            tunnel: w69 -> [w78 w98]
            tunnel: w65 -> [w85 _]
            tunnel: w68 -> [w83 w99]
            tunnel: [w80 w98] -> w67
            tunnel: w63 -> [w79 _]
            tunnel: w62 -> [w74 _]
            frame False {
              # "VISA Name is not empty -> try to connect to the device"
              n20 = Not(x=w74) -> (.not. x?=w73:bool)
              n21 = call <instrlib>:"Initialize.vi"("error in (no error)"=w78, "ID Query (True)"=w73, "VISA resource name"=w75) -> ("error out"=w77:errorcluster, "VISA resource name out"=w76:refnum<visa-resource-name>)  [unwired: 7 in]
              n22 = case shown="Error .." w77 {
                selector: w77 -> [w87 w94]
                tunnel: w76 -> [_ _]
                tunnel: [w87 w93] -> w80
                tunnel: w85 -> [w90 w96]
                tunnel: [w91 w95] -> w82
                tunnel: [T1."Connected" ("Result") T1."Not connected" ("Result")] -> w84
                tunnel: w79 -> [w86 _]
                frame No Error {
                  # "Connection succesfull; update handle with current config and return \"Connected\" as the result"
                  n23 = Bundle By Name(cluster=w90, "Source-meter"=w86, "Connected"=TRUE) -> (w91:T20)
                }
                frame Error {
                  # "Clear connection error"
                  # "Connection failed: set handle and result to \"Not connected\""
                  n24 = call <vilib>:"Clear Errors.vi"("error in (no error)"=w94) -> ("error out"=w93:errorcluster)  [unwired: 5 in, 1 out]
                  n25 = Bundle By Name(cluster=w96, "Connected"=FALSE ("Temp handle.Connected")) -> (w95:T20)
                }
              }
              n26 = Bundle By Name(cluster=w83, "Source-meter handle"=w82) -> (w81:T2)
            }
            frame True {
              # "VISA Name was not provided, return \"Incorrect settings\" as the result"
            }
          }
        }
      }
    }
    frame True {
      # "Controller is already connected"
    }
  }
  "Loop data Out" <- w7
  "Error Out" <- w4
  "Result" <- w6
